vi "Chrg_Dschrg_No_cDAQ.vi"(0 "Strain Gauge":dbl, 2 "Thermocouple":dbl, 4 "PS VISA in":refnum<visa-resource-name>, 5 "PS error in":errorcluster, 6 "DischargeCyclePath":path=path "C:/Users/ga11/Desktop/VI/results/3PtestCharge.lvm" caption="Filename", 8 "Charge/discharge":enum8{"Charge", "Discharge"}(ring), 9 "Charge/Discharge Voltage Setpoint":dbl format="%#.6g", 10 "CC or CCCV":enum16{"CC", "CCCV"}(ring), 11 "Current Setpoint":dbl format="%#.6g", 12 "Output Safety":T1, 13 "Current Cutoff":dbl) -> (18 "PS VIS resource name out":refnum<visa-resource-name>, 19 "PS error out":errorcluster)   [LabVIEW 2020]
uses:
  Drivers-NHR-9200/NHR/Public/Data/Low Level/Fetch (Ave Voltage).vi
  Drivers-NHR-9200/NHR/NH Research Regenerative Test Series.lvlib
panel:
  out "Read Ave Current (A)":dbl
  out "Read Ave Voltage (V)":dbl
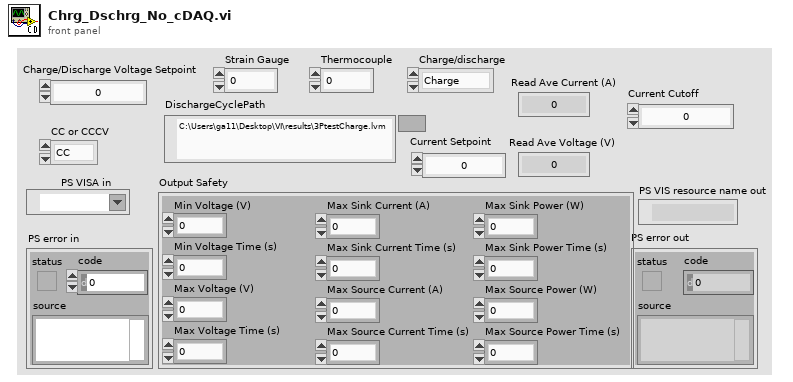
[diagram p1: front panel]
types:
  T1 = cluster{"Min Voltage (V)":dbl, "Min Voltage Time (s)":dbl, "Max Voltage (V)":dbl, "Max Voltage Time (s)":dbl, "Max Sink Current (A)":dbl, "Max Sink Current Time (s)":dbl, "Max Source Current (A)":dbl, "Max Source Current Time (s)":dbl, "Max Sink Power (W)":dbl, "Max Sink Power Time (s)":dbl, "Max Source Power (W)":dbl, "Max Source Power Time (s)":dbl}
  T2 = cluster{"Voltage Enabled":bool, "Current Enabled":bool, "Power Enabled":bool, "Resistance Enabled":bool}
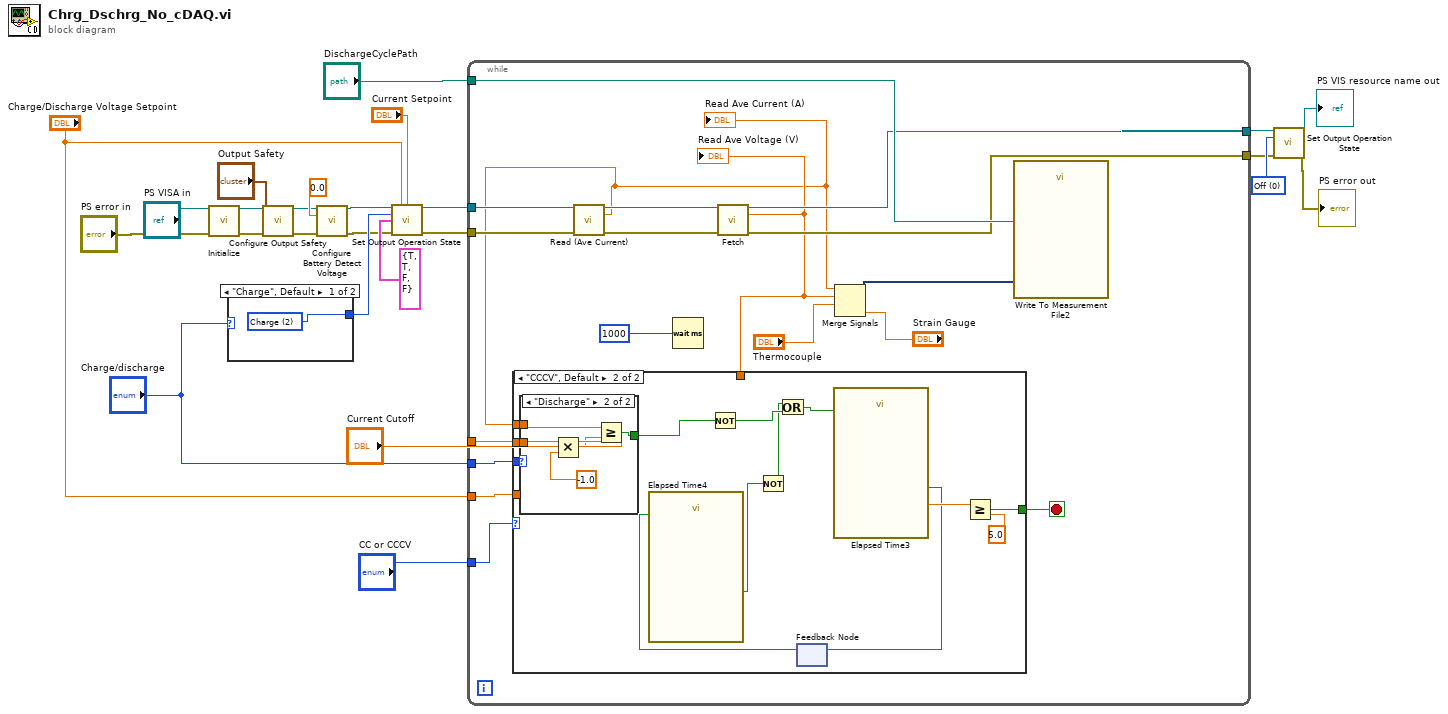
[diagram p0: block diagram]
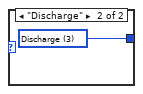
[diagram p2: hidden frame]
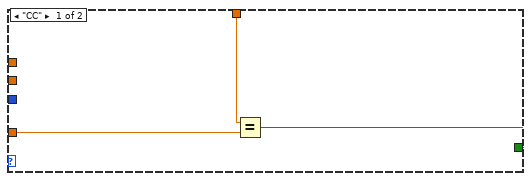
[diagram p3: hidden frame]
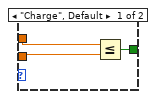
[diagram p4: hidden frame]
diagram:
  w14 = 0 items=["Off", "Standby", "Charge", "Discharge", "Battery"] ("Mode (0: Off)")
  n1 = call "Initialize.vi"("VISA resource name"="PS VISA in", "error in (no error)"="PS error in") -> ("VISA resource name out"=w5:refnum<visa-resource-name>, "error out"=w6:errorcluster)  [unwired: 12 in]
  n2 = case shown="\"Charge\", Default" "Charge/discharge" {
    tunnel: [w26 w27] -> w15
    frame "Charge", Default {
      w26 = 2 items=["Off", "Standby", "Charge", "Discharge", "Battery"] ("Mode (0: Off)")
    }
    frame "Discharge" {
      w27 = 3 items=["Off", "Standby", "Charge", "Discharge", "Battery"] ("Mode (0: Off)")
    }
  }
  n3 = call "Configure Output Safety.vi"("VISA resource name"=w5, "Output Safety"="Output Safety", "error in (no error)"=w6) -> ("VISA resource name out"=w8:refnum<visa-resource-name>, "error out"=w7:errorcluster)  [unwired: 11 in]
  n4 = call "Configure Battery Detect Voltage.vi"("VISA resource name"=w8, "Battery Detect Voltage (0V)"=0.0, "error in (no error)"=w7) -> ("VISA resource name out"=w13:refnum<visa-resource-name>, "error out"=w12:errorcluster)  [unwired: 11 in]
  n5 = call "Set Output Operation State.vi"("VISA resource name"=w13, "Voltage Setpoint (0 V)"="Charge/Discharge Voltage Setpoint", "Current Setpoint (0 A)"="Current Setpoint", "Mode (0: Off)"=w15, "Enable"=T2 {"Voltage Enabled"=TRUE, "Current Enabled"=TRUE, "Power Enabled"=FALSE, "Resistance Enabled"=FALSE}, "error in (no error)"=w12) -> ("VISA resource name out"=w18:refnum<visa-resource-name>, "error out"=w17:errorcluster)  [unwired: 8 in]
  n6 = while {
    tunnel: w18 -> [w32]
    tunnel: w17 -> [w31]
    tunnel: "Current Cutoff" -> [w39]
    tunnel: "DischargeCyclePath" -> [w42]
    tunnel: [w41] -> w10
    tunnel: [w40] -> w9
    tunnel: "CC or CCCV" -> [w38]
    tunnel: "Charge/Discharge Voltage Setpoint" -> [w36]
    tunnel: "Charge/discharge" -> [w35]
    stop <- w43 stop-if-true
    n7 = call "Read (Ave Current).vi"("VISA resource name"=w32, "error in (no error)"=w31) -> ("VISA resource name out"=w29:refnum<visa-resource-name>, "Ave Current (A)"=w28:dbl, "error out"=w30:errorcluster)  [unwired: 11 in]
    "Read Ave Current (A)" <- w28
    n8 = Wait (ms)(milliseconds to wait=1000) -> ()  [unwired: 1 out]
    n9 = call-poly "Fetch.vi"("VISA resource name"=w29, "error in (no error)"=w30) -> ("VISA resource name out"=w41:refnum<visa-resource-name>, "Ave Voltage (V)"=w37:dbl, "error out"=w40:errorcluster)  [unwired: 11 in]
    "Read Ave Voltage (V)" <- w37
    n10 = case shown="\"CCCV\", Default" w38 {
      tunnel: [w46 w55] -> w43
      tunnel: w39 -> [_ w52]
      tunnel: w28 -> [_ w51]
      tunnel: w37 -> [w48 _]
      tunnel: w36 -> [w47 _]
      tunnel: w35 -> [_ w49]
      frame "CC" {
        n11 = Equal?(x=w48, y=w47) -> (x = y?=w46:bool)
      }
      frame "CCCV", Default {
        n12 = case shown="\"Discharge\"" w49 {
          tunnel: w52 -> [w63 w68]
          tunnel: w51 -> [w64 w66]
          tunnel: [w62 w65] -> w50
          frame "Charge", Default {
            n13 = Less Or Equal?(x=w64, y=w63) -> (x <= y?=w62:bool)
          }
          frame "Discharge" {
            n14 = Multiply(x=w68, y=-1.0) -> (x*y=w67:dbl)
            n15 = Greater Or Equal?(x=w66, y=w67) -> (x >= y?=w65:bool)
          }
        }
        n16 = Not(x=w50) -> (.not. x?=w61:bool)
        n17 = feedback #1() -> (w53:bool)  [unwired: 1 in]
        n18 = call "Elapsed Time4"("Reset"=w53) -> ("Time has Elapsed"=w60:bool)  [unwired: 11 in, 7 out]
        n19 = Not(x=w60) -> (.not. x?=w59:bool)
        n20 = Or(x=w59, y=w61) -> (x .or. y?=w58:bool)
        n21 = call "Elapsed Time3"("Reset"=w58) -> ("Elapsed Time (s)"=w57:dbl, "Time has Elapsed"=w54:bool)  [unwired: 11 in, 6 out]
        n22 = feedback-in #1(w54) -> ()
        n23 = Greater Or Equal?(x=w57, y=5.0) -> (x >= y?=w55:bool)
      }
    }
    n24 = Merge Signals "Merge Signals"(w28, w37, "Thermocouple", "Strain Gauge") -> (w45:dynamicdata)
    n25 = call "Write To Measurement File2"("Signals"=w45, "Filename"=w42) -> ()  [unwired: 15 in, 3 out]
  }
  n26 = call "Set Output Operation State.vi"("VISA resource name"=w10, "Mode (0: Off)"=w14, "error in (no error)"=w9) -> ("VISA resource name out"=→"PS VIS resource name out":refnum<visa-resource-name>, "error out"=→"PS error out":errorcluster)  [unwired: 11 in]
